vi "GetBoxNo.vi"(8 "error in":errorcluster caption="错误输入", 9 "种类":enum16{"自产", "外购"}(ring), 10 "TimeStr":string, 11 "Model":string) -> (0 "error out":errorcluster caption="错误输出", 3 "BoxNo":string)   [LabVIEW 2013]
panel:
  out "最大值":string
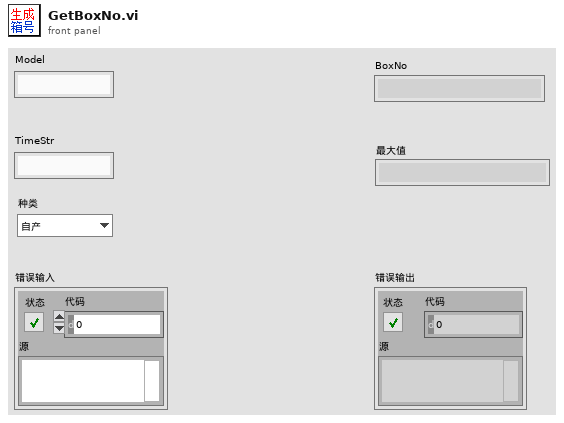
[diagram p1: front panel]
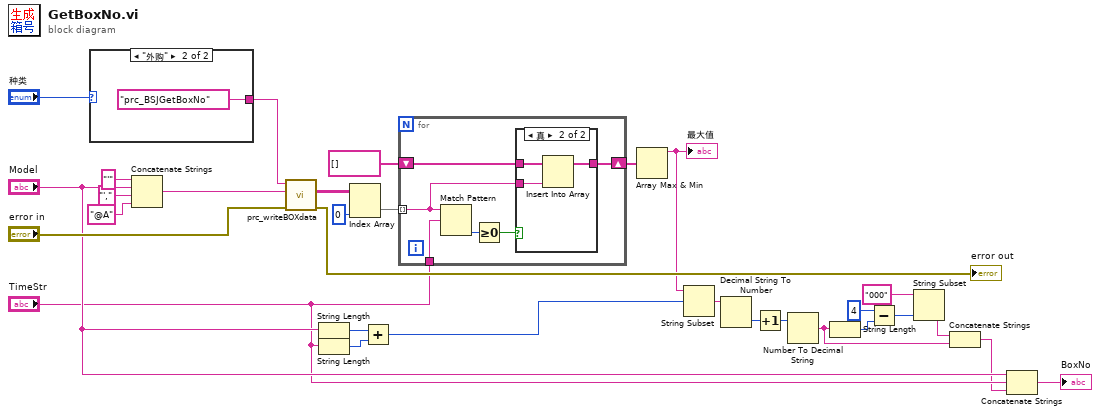
[diagram p0: block diagram]
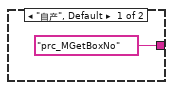
[diagram p2: hidden frame]
diagram:
  n1 = case shown="\"外购\"" "种类" {
    tunnel: ["prc_MGetBoxNo" ("Process") "prc_BSJGetBoxNo" ("Process")] -> w30
    frame "自产", Default {
    }
    frame "外购" {
    }
  }
  n2 = Concatenate Strings("'", "Model", "',", "@A" ("字符串")) -> (w26:string)
  n3 = call "prc_writeBOXdata.vi"("error in"="error in", "string"=w26, "Process"=w30) -> ("error out"=→"error out":errorcluster, "Array"=w24:string[][])  [unwired: 7 in]
  n4 = String Length(string="Model") -> (length=w16:i32)
  n5 = String Length(string="TimeStr") -> (length=w17:i32)
  n6 = Index Array(array=w24, index (col)=0 ("禁用的索引 (列)")) -> (element=w23:string[])  [unwired: 1 in]
  n7 = Add(x=w16, y=w17) -> (x+y=w15:i32)
  n8 = for {
    tunnel: w23 -> [w34] mode=indexing
    shift-right: [w33] -> w21
    shift-left: string[] [] ("子数组") -> [w35]
    tunnel: "TimeStr" -> [w38]
    n9 = Match Pattern(string=w34, regular expression=w38) -> (offset past match=w37:i32)  [unwired: 1 in, 3 out]
    n10 = Greater Or Equal To 0?(x=w37) -> (x >= 0?=w36:bool)
    n11 = case shown="真" w36 {
      tunnel: w35 -> [w39 w42]
      tunnel: w34 -> [_ w41]
      tunnel: [w39 w40] -> w33
      frame False {
      }
      frame True {
        n12 = Insert Into Array(array=w42, new element=w41) -> (w40:string[])  [unwired: 1 in]
      }
    }
  }
  n13 = Array Max & Min(array=w21) -> (max value=w18:string)  [unwired: 3 out]
  "最大值" <- w18
  n14 = String Subset(string=w18, offset (0)=w15) -> (substring=w12:string)  [unwired: 1 in]
  n15 = Decimal String To Number(string=w12) -> (number=w11:i32)  [unwired: 2 in, 1 out]
  n16 = Increment(x=w11) -> (x+1=w10:i32)
  n17 = Number To Decimal String(number=w10) -> (decimal integer string=w3:string)  [unwired: 1 in]
  n18 = String Length(string=w3) -> (length=w7:i32)
  n19 = Subtract(x=4, y=w7) -> (x-y=w6:i32)
  n20 = String Subset(string="000", length (rest)=w6) -> (substring=w4:string)  [unwired: 1 in]
  n21 = Concatenate Strings(w4, w3) -> (w2:string)
  n22 = Concatenate Strings("Model", "TimeStr", w2) -> (→"BoxNo":string)
